vi "ApproximatelyEqualFunction.vi"(9 "Margin":dbl, 10 "Setpoint":dbl, 11 "Variable":dbl) -> (3 "t/f":bool)   [LabVIEW 2017]
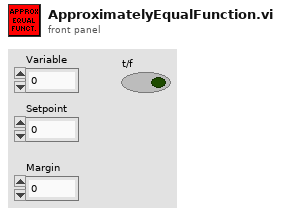
[diagram p1: front panel]
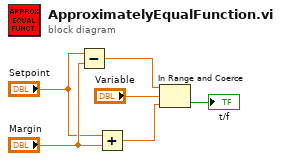
[diagram p0: block diagram]
diagram:
  n1 = Subtract(x="Setpoint", y="Margin") -> (x-y=w3:dbl)
  n2 = Add(x="Setpoint", y="Margin") -> (x+y=w2:dbl)
  n3 = In Range and Coerce(upper limit=w3, x="Variable", lower limit=w2) -> (In Range?=→"t/f":bool)  [unwired: 1 out]
